vi "wybierz typ kursora.vi"(6 "Swobodny":i32, 9 "Plot in":i32, 10 "Cursor Mode":u32, 11 "Plots in":i32[](array[numeric])) -> (2 "Plot2 out":i32, 3 "Plot1 out":i32)   [LabVIEW 2014]
doc: "Wybiera typ swobodny jeœli cursor mode 0"
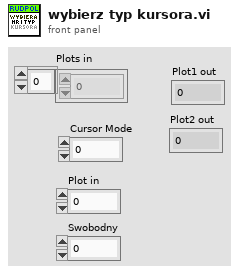
[diagram p1: front panel]
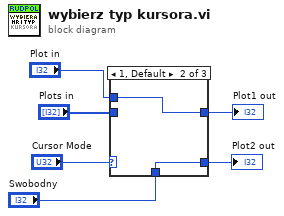
[diagram p0: block diagram]
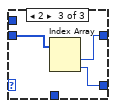
[diagram p3: hidden frame]
diagram:
  n1 = case shown="1, Default" "Cursor Mode" {
    tunnel: "Plots in" -> [_ _ w12]
    tunnel: [w7 w8 w11] -> w6
    tunnel: "Swobodny" -> [w7 w9 _]
    tunnel: [w7 w9 w10] -> w3
    tunnel: "Plot in" -> [_ w8 _]
    frame 0 {
    }
    frame 1, Default {
    }
    frame 2 {
      n2 = Index Array(array=w12) -> (element #1=w11:i32, element #2=w10:i32)  [unwired: 2 in]
    }
  }
  "Plot1 out" <- w6
  "Plot2 out" <- w3
